vi "Set Saturation Event.vi"(11 "saturationEvent":u32) -> (2 "function return":u32, 3 "saturationEvent out":u32)   [LabVIEW 2018, in "AndorSDK.lvlib"]
doc: "EXPNETTYPE unsigned int WINAPI SetSaturationEvent(HANDLE saturationEvent);"
uses:
  AndorSDK.lvlib
  ATMCD32D.dll
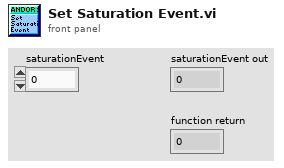
[diagram p1: front panel]
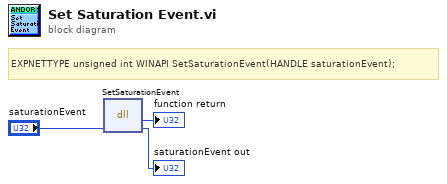
[diagram p0: block diagram]
diagram:
  # "EXPNETTYPE unsigned int WINAPI SetSaturationEvent(HANDLE saturationEvent);"
  n1 = dll-call lib="PTH2babs E\nPersönliches02 - Arbeit03-HiwijobsLabviewCodelibANDOR\tAndor SDK\nATMCD32D.*" fn="SetSaturationEvent"("saturationEvent"="saturationEvent") -> (→"function return":u32, "saturationEvent"=→"saturationEvent out":u32)  [unwired: 3 in, 2 out]
